vi "Close KUKA youBot.vi"(8 "error in (no error)":errorcluster, 11 "KUKA youBot host in":refnum<class "NI_Robotics_KUKA youBot Host_EtherCAT.lvclass">) -> (0 "error out":errorcluster)   [LabVIEW 2017, in "NI_Robotics_KUKA youBot Host.lvlib" / "NI_Robotics_KUKA youBot Host_EtherCAT.lvclass"]
uses:
  <vilib>/robotics/KUKA youBot/EtherCAT Host Interface/NI_Robotics_KUKA youBot Host_EtherCAT.lvclass
  c:/Program Files (x86)/National Instruments/LabVIEW 2017/vi.lib/robotics/KUKA youBot/Host Interface/NI_Robotics_KUKA youBot Host Interface.lvclass
  <vilib>/robotics/KUKA youBot/Host Interface/NI_Robotics_KUKA youBot Host Interface.lvclass/NI_Robotics_KUKA youBot Host Interface.ctl
  <vilib>/robotics/KUKA youBot/Basic Device/Mobile Platform/NI_Robotics_KUKA youBot Platform.lvclass
  <vilib>/robotics/KUKA youBot/Host Interface/NI_Robotics_KUKA youBot Host Interface.lvclass
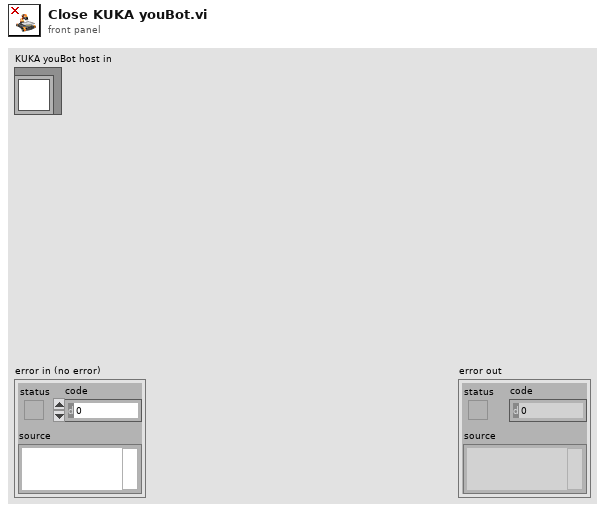
[diagram p1: front panel]
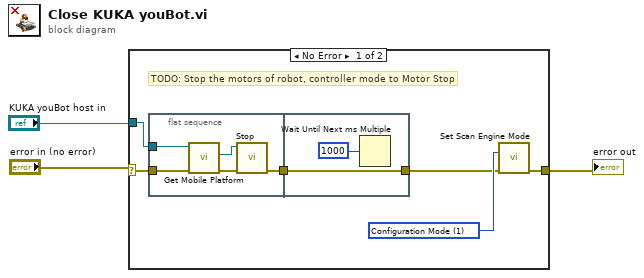
[diagram p0: block diagram]
diagram:
  n1 = case shown="No Error" "error in (no error)" {
    selector: "error in (no error)" -> [w6 w17]
    tunnel: [w8 w17] -> w1
    tunnel: "KUKA youBot host in" -> [w4 _]
    frame No Error {
      w9 = 1 items=["Configuration Mode"=1, "Active Mode"=2] ("mode (Active Mode)")
      # "TODO: Stop the motors of robot, controller mode to Motor Stop"
      n2 = flat-sequence {
        tunnel: w6 -> [w13]
        tunnel: [w10] -> w5
        tunnel: w4 -> [w14]
        tunnel: [w15] -> w7
        tunnel: w5 -> [w15]
        frame #0 {
          n3 = call <vilib>:"Get Mobile Platform.vi"("error in (no error)"=w13, "KUKA youBot host in"=w14) -> ("error out"=w12:errorcluster, "KUKA youBot platform out"=w11:refnum<class "NI_Robotics_KUKA youBot Platform.lvclass">)  [unwired: 7 in, 1 out]
          n4 = call-dynamic "Stop.vi"("error in (no error)"=w12, "KUKA youBot platform in"=w11) -> ("error out"=w10:errorcluster)  [unwired: 8 in, 1 out]
        }
        frame #1 {
          n5 = Wait Until Next ms Multiple(millisecond multiple=u32 1000) -> ()  [unwired: 1 out]
        }
      }
      n6 = call <vilib>:"Set Scan Engine Mode.vi"("mode (Active Mode)"=w9, "error in (no error)"=w7) -> ("error out"=w8:errorcluster)  [unwired: 13 in]
    }
    frame Error {
    }
  }
  "error out" <- w1
